vi "Get VI Members from Path.vi"(2 "error in (no error)":errorcluster, 3 "VI Path":path) -> (0 "error out":errorcluster, 1 "VI Members":path[](array[path]))   [LabVIEW 2009, in "GraphicalTestRunner.lvlib"]
uses:
  GraphicalTestRunner.lvlib
panel:
  in  "application reference (local)":refnum<vi>
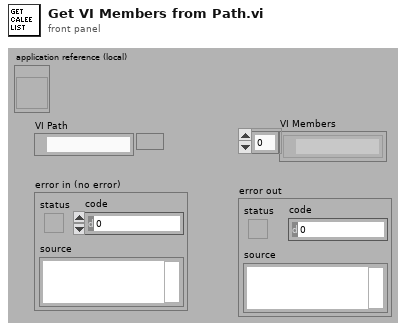
[diagram p1: front panel]
types:
  T1 = typedef "Liner Info - Cluster__jki_lib_application_control.ctl" = cluster{"path":path, "type":enum32{"Instrument", "Control", "CIN", "External subroutine", "Shared library", "Run-time menu", "Help file", "Palette menu"}, "iState":u32, "iStyle":u16, "wStyle":u16, "buttons":u16, "viflags":u32, "viflags2":u32, "links":u32[]}
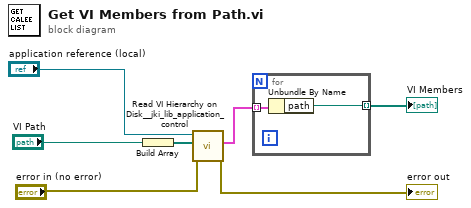
[diagram p0: block diagram]
diagram:
  n1 = Build Array("VI Path") -> (w6:path[])
  n2 = call <vilib>:"Read VI Hierarchy on Disk__jki_lib_application_control.vi"("error in"="error in (no error)", "Paths to Read"=w6, "application reference (local)"="application reference (local)") -> ("error out"=→"error out":errorcluster, "Linker Info"=w2:T1[])  [unwired: 5 in, 2 out]
  n3 = for {
    tunnel: w2 -> [w9] mode=indexing
    tunnel: [w8] -> w1 mode=indexing
    n4 = Unbundle By Name(w9) -> ("path"=w8:path)
  }
  "VI Members" <- w1
